vi "ziCpuProgram.vi"(3 "error in":errorcluster, 4 "device (active)":string, 5 "Filename":string, 6 "Handle In":T1 {"Handle" format="0x%08x"; "Conn" format="0x%08x"}) -> (0 "error out":errorcluster, 2 "Handle Out":T1 {"Handle" format="0x%08x"; "Conn" format="0x%08x"})   [LabVIEW 2018, in "Zurich Instruments LabOne.lvlib"]
doc: "This vi programs the RT option of an HF2 Series instrument"
uses:
  Zurich Instruments LabOne.lvlib
  <instrlib>/Zurich Instruments LabOne/Private/ziLV64.framework
  ziTypeHandle.ctl
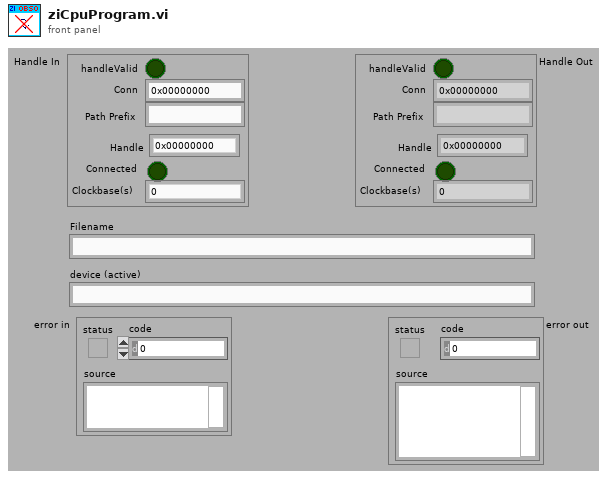
[diagram p1: front panel]
types:
  T1 = typedef "Zurich Instruments LabOne.lvlib/ziTypeHandle.ctl" = cluster{"handleValid":bool, "Conn":u64, "Path Prefix":string, "Handle":u64, "Connected":bool, "Clockbase(s)":dbl}
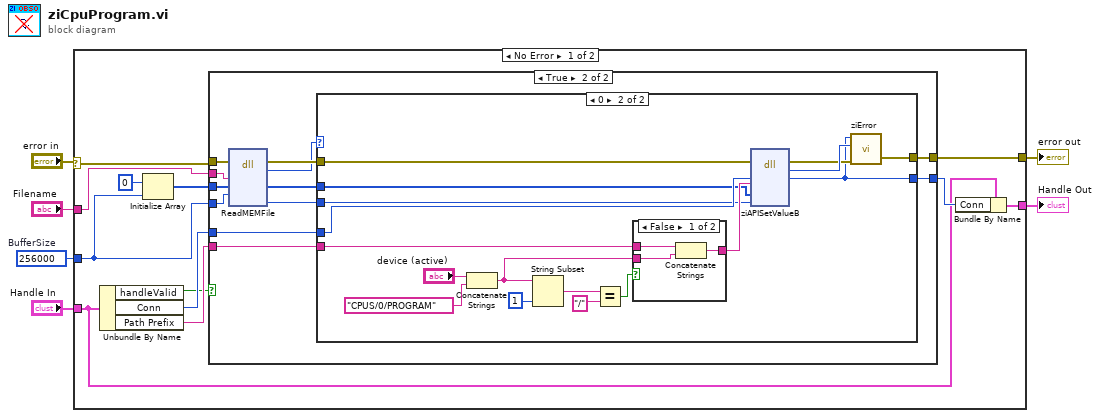
[diagram p0: block diagram]
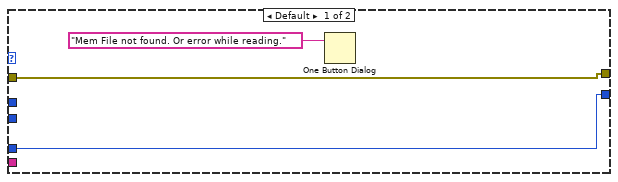
[diagram p3: hidden frame]
diagram:
  w4 = 256000  # BufferSize
  n1 = case shown="No Error" "error in" {
    selector: "error in" -> [w7 w57]
    tunnel: [w18 w57] -> w6
    tunnel: "Filename" -> [w16 _]
    tunnel: w4 -> [w12 _]
    tunnel: [w9 w58] -> w3
    tunnel: "Handle In" -> [w8 w58]
    frame No Error {
      n2 = Unbundle By Name(w8) -> ("handleValid"=w13:bool, "Conn"=w15:u64, "Path Prefix"=w17:string)
      n3 = Initialize Array(u8 0 ("element"), w12) -> (w10:u8[])
      n4 = case shown="True" w13 {
        tunnel: w7 -> [w19 w32]
        tunnel: w12 -> [_ w31]
        tunnel: [w19 w30] -> w18
        tunnel: w17 -> [_ w29]
        tunnel: w16 -> [_ w28]
        tunnel: w15 -> [w20 w26]
        tunnel: [w20 w23] -> w14
        tunnel: w10 -> [_ w21]
        frame False {
        }
        frame True {
          n5 = dll-call lib="Applications/National Instruments/LabVIEW 2019 64-bit/instr.lib/Zurich Instruments LabOne/Private/ziLV*.*" fn="ReadMEMFile"(error in=w32, "Filename"=w28, "Buffer"=w21, "BuffeSize"=w31) -> (error out=w27:errorcluster, "return type"=w22:u32, "Buffer"=w25:u8[], "bytesUsed"=w24:u32)  [unwired: 4 in, 2 out]
          n6 = case shown="0" w22 {
            tunnel: [w33 w52] -> w30
            tunnel: w29 -> [_ w47]
            tunnel: w27 -> [w33 w46]
            tunnel: w26 -> [w35 w44]
            tunnel: w25 -> [_ w43]
            tunnel: w24 -> [_ w42]
            tunnel: [w35 w36] -> w23
            frame Default {
              n7 = One Button Dialog(message="Mem File not found. Or error while reading.") -> ()  [unwired: 2 out]
            }
            frame 0 {
              n8 = Concatenate Strings("device (active)", "CPUS/0/PROGRAM") -> (w37:string)
              n9 = String Subset(string=w37, length (rest)=1 ("length (rest)")) -> (substring=w50:string)  [unwired: 1 out]
              n10 = Equal?(x=w50, y="/") -> (x = y?=w48:bool)
              n11 = case shown="False" w48 {
                tunnel: w47 -> [w53 _]
                tunnel: [w55 w56] -> w45
                tunnel: w37 -> [w54 w56]
                frame False {
                  n12 = Concatenate Strings(w53, w54) -> (w55:string)
                }
                frame True {
                }
              }
              n13 = dll-call lib="Applications/National Instruments/LabVIEW 2019 64-bit/instr.lib/Zurich Instruments LabOne/Private/ziLV*.*" fn="ziAPISetValueB"(error in=w46, "Conn"=w44, "Path"=w45, "Buffer"=w43, "Len"=w42) -> (error out=w40:errorcluster, "return type"=w41:u32, "Conn"=w36:u64)  [unwired: 5 in, 1 out]
              n14 = call "ziError.vi"("Conn"=w36, "ziErrorCode"=w41, "Error In"=w40) -> ("Error Out"=w52:errorcluster)  [unwired: 2 in, 1 out]
            }
          }
        }
      }
      n15 = Bundle By Name(cluster=w8, "Conn"=w14) -> (w9:T1)
    }
    frame Error {
    }
  }
  "error out" <- w6
  "Handle Out" <- w3
